vi "Model--Order Key Values.vi"(8 "error in":errorcluster, 10 "KVP In":cluster{"Name":string, "Value":variant}[](array[cluster]), 11 "Selector in":refnum<class "Selector.lvclass">) -> (0 "error out":errorcluster, 2 "KVP Out":cluster{"Name":string, "Value":variant}[](array[cluster]), 3 "Selector out":refnum<class "Selector.lvclass">)   [LabVIEW 2019, in "Selector.lvclass"]
uses:
  Selector.lvclass
  Selector.lvclass/Selector.ctl
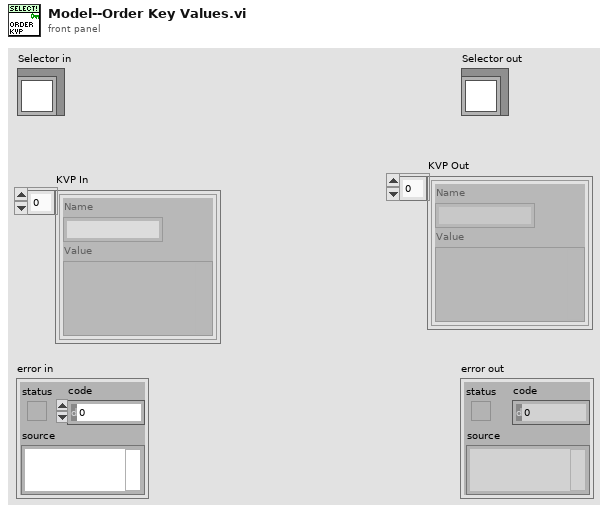
[diagram p1: front panel]
types:
  T1 = cluster{"Name":string, "Group":string, "Enabled":bool}[]
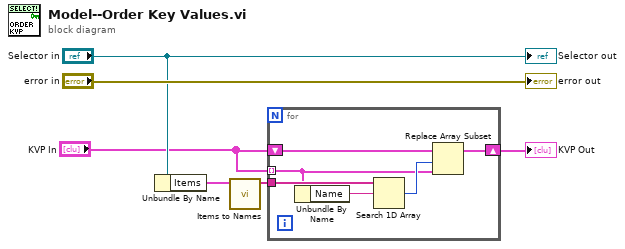
[diagram p0: block diagram]
diagram:
  n1 = Unbundle By Name("Selector in") -> ("Items"=w1:T1)
  n2 = call "Items to Names.vi"("Items"=w1) -> ("Names"=w4:string[])  [unwired: 6 in]
  n3 = for {
    tunnel: w4 -> [w12]
    tunnel: "KVP In" -> [w8] mode=indexing
    shift-right: [w7] -> w3
    shift-left: "KVP In" -> [w10]
    n4 = Unbundle By Name(w8) -> ("Name"=w11:string)
    n5 = Search 1D Array(1D array=w12, element=w11) -> (index of element=w9:i32)  [unwired: 1 in]
    n6 = Replace Array Subset(array=w10, new element=w8, index=w9) -> (w7:cluster{"Name":string, "Value":variant}[])
  }
  "KVP Out" <- w3
  "error out" <- "error in"
  "Selector out" <- "Selector in"
